vi "new_table.vi"(8 "error in (no error)":errorcluster) -> (0 "error out":errorcluster, 3 "Table out":refnum<class "Table.lvclass">)   [LabVIEW 2020, in "toml_edit.lvlib" / "Table.lvclass"]
uses:
  Table.lvclass
  Table.lvclass/Table.ctl
  dragon_toml_64.dll
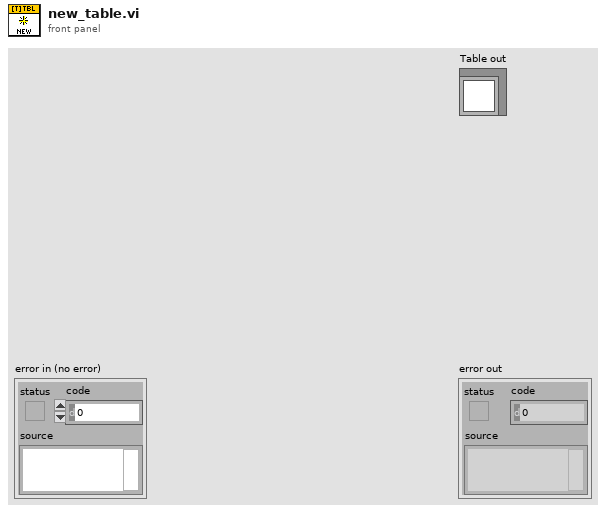
[diagram p1: front panel]
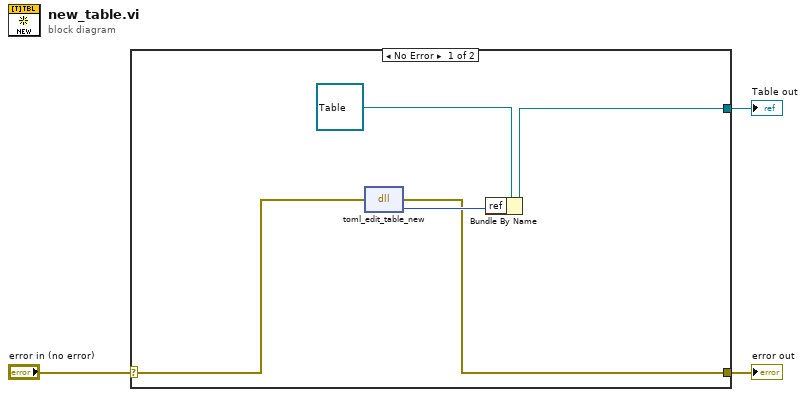
[diagram p0: block diagram]
diagram:
  n1 = case shown="No Error" "error in (no error)" {
    selector: "error in (no error)" -> [w5 w9]
    tunnel: [w4 w9] -> w2
    tunnel: [w6 _] -> w1
    frame No Error {
      n2 = dll-call lib="C:/projects/dragon-desktop/source/submodules/toml-edit-labview/lv_src/dragon_toml_*.*" fn="toml_edit_table_new"(error in=w5) -> (error out=w4:errorcluster, "table"=w8:u64)  [unwired: 2 in, 1 out]
      n3 = Bundle By Name(cluster=refnum<class "Table.lvclass"> refnum ("Table out"), "ref"=w8) -> (w6:refnum<class "Table.lvclass">)
    }
    frame Error {
    }
  }
  "error out" <- w2
  "Table out" <- w1
